vi "PZT Set Position.vi"(8 "error in (no error)":errorcluster caption="错误输入（无错误）", 9 "电压值（V）":i32, 10 "Set Position （°/mm）":dbl, 11 "VISA resource name":refnum<visa-resource-name> caption="VISA资源名称") -> (0 "错误输出":errorcluster, 2 "Current Position （°/mm）":dbl, 3 "VISA resource name 2":refnum<visa-resource-name>)   [LabVIEW 2014]
uses:
  Global Para.vi
panel:
  out "Steps calculated":i32
  out "Steps left":i32
  in  "step size (mm)":dbl=0.0001
  in  "critical value (mm)":dbl=0.002
  out "Goal":bool
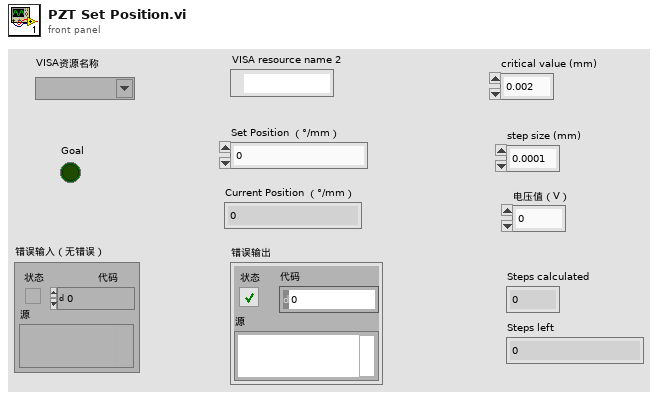
[diagram p1: front panel]
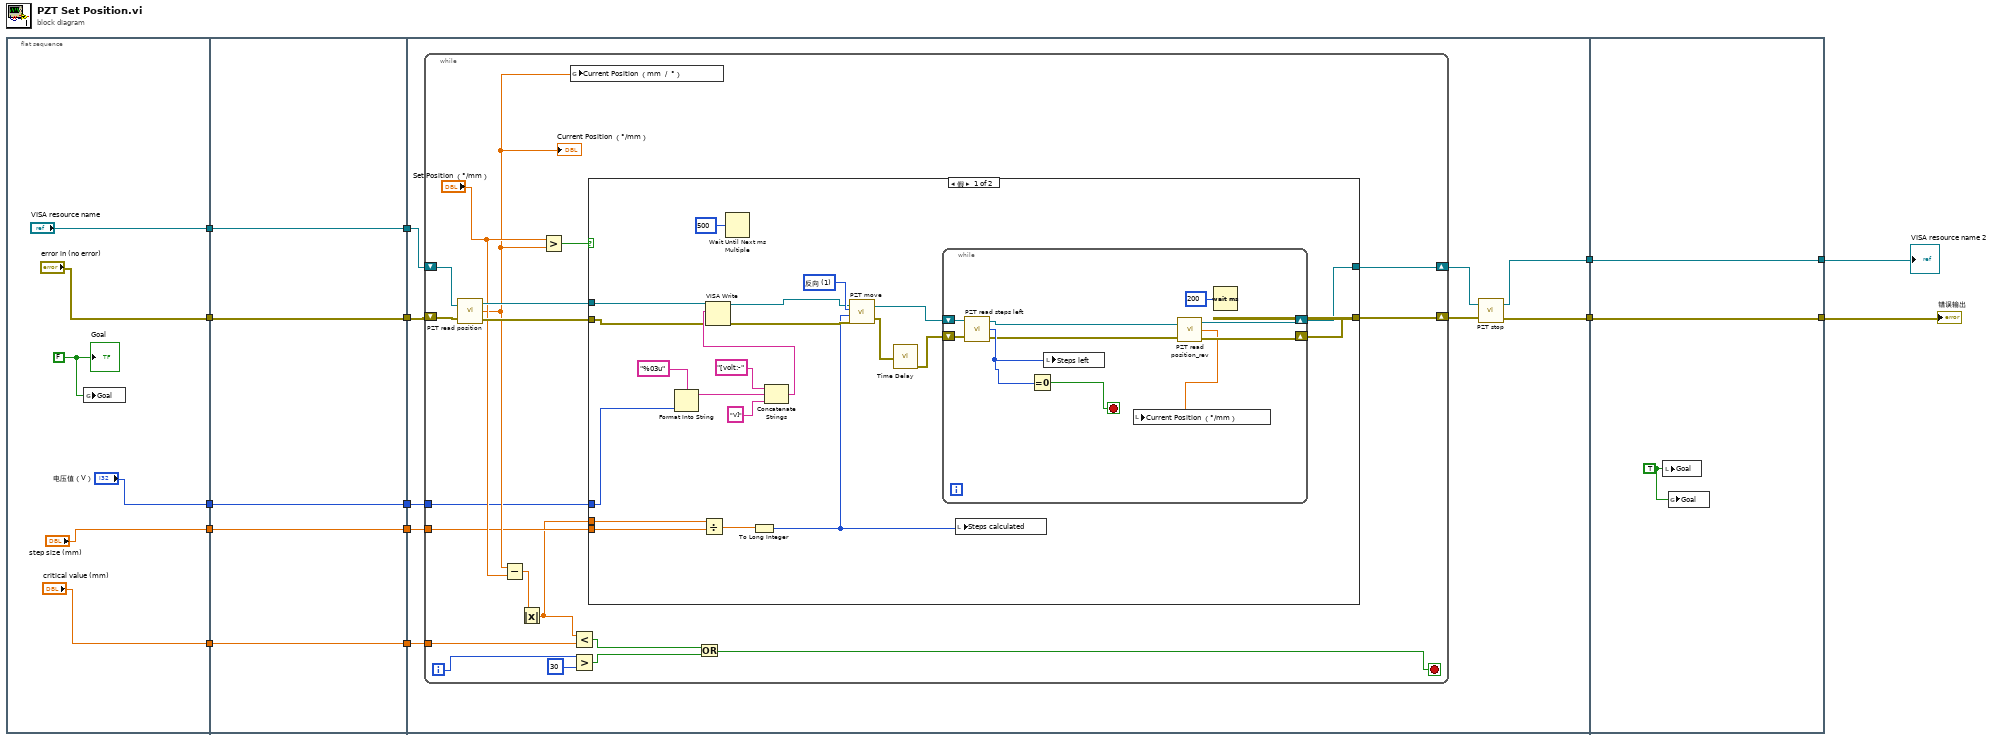
[diagram p0: block diagram]
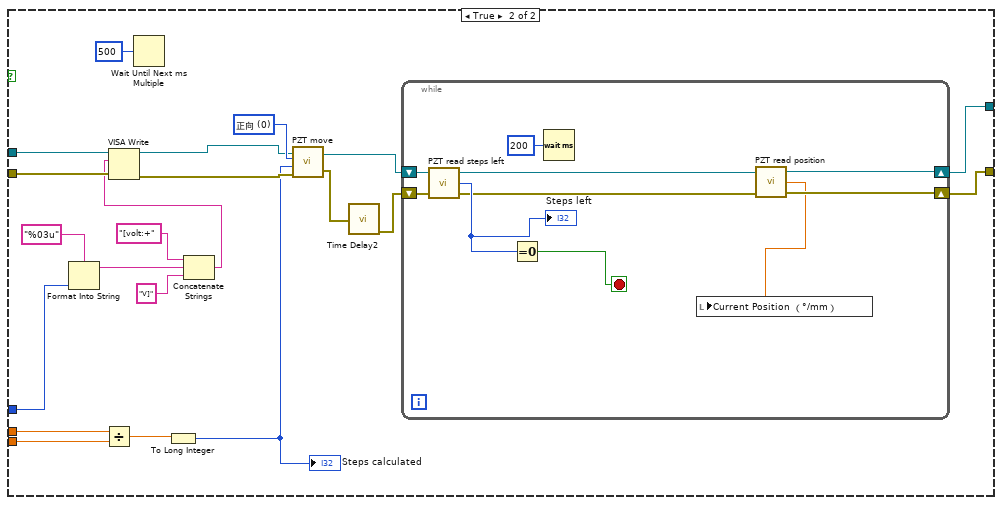
[diagram p2: hidden frame]
diagram:
  n1 = flat-sequence {
    tunnel: ["VISA resource name"] -> w12
    tunnel: ["error in (no error)"] -> w9
    tunnel: ["critical value (mm)"] -> w5
    tunnel: ["电压值（V）"] -> w3
    tunnel: ["step size (mm)"] -> w1
    tunnel: w12 -> [w25]
    tunnel: [w25] -> w11
    tunnel: [w24] -> w10
    tunnel: w9 -> [w24]
    tunnel: [w23] -> w6
    tunnel: w5 -> [w23]
    tunnel: [w22] -> w4
    tunnel: w3 -> [w22]
    tunnel: [w21] -> w2
    tunnel: w1 -> [w21]
    tunnel: [w29] -> w14
    tunnel: [w32] -> w13
    tunnel: w11 -> [w30]
    tunnel: w10 -> [w31]
    tunnel: w6 -> [w28]
    tunnel: w4 -> [w27]
    tunnel: w2 -> [w26]
    tunnel: [w117] -> w7
    tunnel: [w118] -> w8
    tunnel: w14 -> [w118]
    tunnel: w13 -> [w117]
    frame #0 {
      w20 = FALSE ("Goal")
      n2 = global write "Global Para.vi" "Goal"(w20) -> ()
      "Goal" <- w20
    }
    frame #1 {
    }
    frame #2 {
      n3 = while {
        shift-right: [w50] -> w34
        shift-left: w31 -> [w48]
        shift-right: [w49] -> w33
        shift-left: w30 -> [w47]
        tunnel: w28 -> [w46]
        tunnel: w27 -> [w38]
        tunnel: w26 -> [w36]
        i -> [w42]
        stop <- w39 stop-if-true
        n4 = call "PZT read position.vi"("VISA resource name"=w47, "error in (no error)"=w48) -> ("VISA资源名称输出"=w52:refnum<visa-resource-name>, "Current Position （mm  /  °）"=w44:dbl, "错误输出"=w51:errorcluster)
        "Current Position （°/mm）" <- w44
        n5 = Subtract(x=w44, y="Set Position （°/mm）") -> (x-y=w37:dbl)
        n6 = Absolute Value(x=w37) -> (abs(x)=w35:dbl)
        n7 = Greater?(x="Set Position （°/mm）", y=w44) -> (0:w53:bool)
        n8 = global write "Global Para.vi" "Current Position （mm  /  °）"(w44) -> ()
        n9 = Less?(x=w35, y=w46) -> (x < y?=w43:bool)
        n10 = Greater?(x=w42, y=30) -> (0:w40:bool)
        n11 = case shown="假" w53 {
          tunnel: w52 -> [w58 w94]
          tunnel: w51 -> [w57 w93]
          tunnel: [w56 w105] -> w49
          tunnel: [w55 w104] -> w50
          tunnel: w38 -> [w59 w90]
          tunnel: w35 -> [w61 w88]
          tunnel: w36 -> [w60 w87]
          frame False {
            w74 = u16 1 items=["正向", "反向"] ("移动方向")
            n12 = Format Into String(format string="%03u" ("格式字符串"), w59) -> (resulting string=w68:string)  [unwired: 2 in, 1 out]
            n13 = Divide(x=w61, y=w60) -> (x/y=w62:dbl)
            n14 = Wait Until Next ms Multiple(millisecond multiple=u32 500) -> ()  [unwired: 1 out]
            n15 = To Long Integer(number=w62) -> (32bit integer=w54:i32)
            n16 = Concatenate Strings("[volt:-" ("字符串"), w68, "V]" ("字符串")) -> (w63:string)
            n17 = VISA Write(VISA resource name=w58, write buffer=w63, error in (no error)=w57) -> (VISA resource name out=w65:refnum<visa-resource-name>, error out=w64:errorcluster)  [unwired: 1 out]
            n18 = call "PZT move.vi"("error in (no error)"=w64, "移动步数"=w54, "移动方向"=w74, "VISA resource name"=w65) -> ("错误输出"=w71:errorcluster, "VISA资源名称输出"=w73:refnum<visa-resource-name>)
            n19 = call "Time Delay"("error in (no error)"=w71) -> ("error out"=w70:errorcluster)  [unwired: 10 in]
            n20 = while {
              shift-right: [w77] -> w56
              shift-left: w73 -> [w84]
              shift-right: [w76] -> w55
              shift-left: w70 -> [w83]
              stop <- w82 stop-if-true
              n21 = call "PZT read steps left.vi"("VISA resource name"=w84, "error in (no error)"=w83) -> ("VISA资源名称输出"=w79:refnum<visa-resource-name>, "Steps left"=w80:i32, "错误输出"=w78:errorcluster)
              n22 = Equal To 0?(x=w80) -> (x = 0?=w82:bool)
              n23 = local write "Steps left"(w80) -> ()
              n24 = call "PZT read position_rev.vi"("VISA resource name"=w79, "error in (no error)"=w78) -> ("VISA资源名称输出"=w77:refnum<visa-resource-name>, "Current Position （mm  /  °）"=w75:dbl, "错误输出"=w76:errorcluster)
              n25 = local write "Current Position （°/mm）"(w75) -> ()
              n26 = Wait (ms)(milliseconds to wait=u32 200 ("等待时间（毫秒）")) -> ()  [unwired: 1 out]
            }
            n27 = local write "Steps calculated"(w54) -> ()
          }
          frame True {
            w103 = u16 0 items=["正向", "反向"] ("移动方向")
            n28 = Format Into String(format string="%03u" ("格式字符串"), w90) -> (resulting string=w97:string)  [unwired: 2 in, 1 out]
            n29 = Divide(x=w88, y=w87) -> (x/y=w86:dbl)
            n30 = Wait Until Next ms Multiple(millisecond multiple=u32 500) -> ()  [unwired: 1 out]
            n31 = To Long Integer(number=w86) -> (32bit integer=w85:i32)
            "Steps calculated" <- w85
            n32 = Concatenate Strings("[volt:+" ("字符串"), w97, "V]" ("字符串")) -> (w89:string)
            n33 = VISA Write(VISA resource name=w94, write buffer=w89, error in (no error)=w93) -> (VISA resource name out=w92:refnum<visa-resource-name>, error out=w91:errorcluster)  [unwired: 1 out]
            n34 = call "PZT move.vi"("error in (no error)"=w91, "移动步数"=w85, "移动方向"=w103, "VISA resource name"=w92) -> ("错误输出"=w100:errorcluster, "VISA资源名称输出"=w102:refnum<visa-resource-name>)
            n35 = call "Time Delay2"("error in (no error)"=w100) -> ("error out"=w99:errorcluster)  [unwired: 10 in]
            n36 = while {
              shift-right: [w110] -> w105
              shift-left: w102 -> [w115]
              shift-right: [w109] -> w104
              shift-left: w99 -> [w114]
              stop <- w113 stop-if-true
              n37 = call "PZT read steps left.vi"("VISA resource name"=w115, "error in (no error)"=w114) -> ("VISA资源名称输出"=w108:refnum<visa-resource-name>, "Steps left"=w111:i32, "错误输出"=w107:errorcluster)
              "Steps left" <- w111
              n38 = Equal To 0?(x=w111) -> (x = 0?=w113:bool)
              n39 = Wait (ms)(milliseconds to wait=u32 200 ("等待时间（毫秒）")) -> ()  [unwired: 1 out]
              n40 = call "PZT read position.vi"("VISA resource name"=w108, "error in (no error)"=w107) -> ("VISA资源名称输出"=w110:refnum<visa-resource-name>, "Current Position （mm  /  °）"=w106:dbl, "错误输出"=w109:errorcluster)
              n41 = local write "Current Position （°/mm）"(w106) -> ()
            }
          }
        }
        n42 = Or(x=w43, y=w40) -> (x .or. y?=w39:bool)
      }
      n43 = call "PZT stop.vi"("error in (no error)"=w34, "VISA resource name"=w33) -> ("错误输出"=w29:errorcluster, "VISA资源名称输出"=w32:refnum<visa-resource-name>)
    }
    frame #3 {
      w116 = TRUE ("Goal")
      n44 = local write "Goal"(w116) -> ()
      n45 = global write "Global Para.vi" "Goal"(w116) -> ()
    }
  }
  "错误输出" <- w8
  "VISA resource name 2" <- w7
